vi "Shooter RPM Testing.vi"   [LabVIEW 2019]
uses:
  <vilib>/Rock Robotics/WPI/ThirdParty/REV Robotics/SPARK MAX/Typedef/Spark MAX Control Type.ctl
  Robot Global Data.vi
  <vilib>/Analysis/NI_AALPro.lvlib
types:
  T1 = typedef "WPI_MotorControlDeviceRef.ctl" = cluster{"DeviceStatus":errorcluster, "Type":T2, "PWM":cluster{"PWM Channel":T3, "DeadBand":T4}, "CAN":cluster{"Device Number":u8, "SetOutput VI Ref":variant, "GetOutput VI Ref":variant, "Enable VI Ref":variant, "Disable VI Ref":variant, "Data":variant}, "Invert":bool, "DIO PWM":cluster{"PWM \"Enable\" Channel":T3, "DIOChannel":T5, "PWM Rate":dbl}}
  T2 = typedef "WPI_MotorControlType.ctl" = enum16{"PWM", "CAN", "DIO PWM"}
  T3 = typedef "FPGA_DIOPWMChannel.ctl" = enum8{"PWM 0", "PWM 1", "PWM 2", "PWM 3", "PWM 4", "PWM 5", "PWM 6", "PWM 7", "PWM 8", "PWM 9", "PWM MXP 0", "PWM MXP 1", "PWM MXP 2", "PWM MXP 3", "PWM MXP 4", "PWM MXP 5", "PWM MXP 6", "PWM MXP 7", "PWM MXP 8", "PWM MXP 9", "Invalid"}
  T4 = typedef "WPI_PWMDeadband.ctl" = cluster{"Name":string, "maxPositivePwm":i32, "minPositivePwm":i32, "centerPwm":i32, "maxNegativePwm":i32, "minNegativePwm":i32, "angularRange":u16}
  T5 = typedef "FPGA_DIOChannel.ctl" = enum8{"DIO 0", "DIO 1", "DIO 2", "DIO 3", "DIO 4", "DIO 5", "DIO 6", "DIO 7", "DIO 8", "DIO 9", "DIO MXP 0", "DIO MXP 1", "DIO MXP 2", "DIO MXP 3", "DIO MXP 4", "DIO MXP 5", "DIO MXP 6", "DIO MXP 7", "DIO MXP 8", "DIO MXP 9", "DIO MXP 10", "DIO MXP 11", "DIO MXP 12", "DIO MXP 13", "DIO MXP 14", "DIO MXP 15", "SPI Port CS1", "SPI Port CS2", "SPI Port CS3", "SPI Port MISO", "SPI Port MOSI", "Invalid"}
  T6 = typedef "Spark MAX Control Type.ctl" = enum16{"Percent VBus", "Voltage", "Velocity", "Position", "Smart Motion", "Current", "Smart Velocity"}
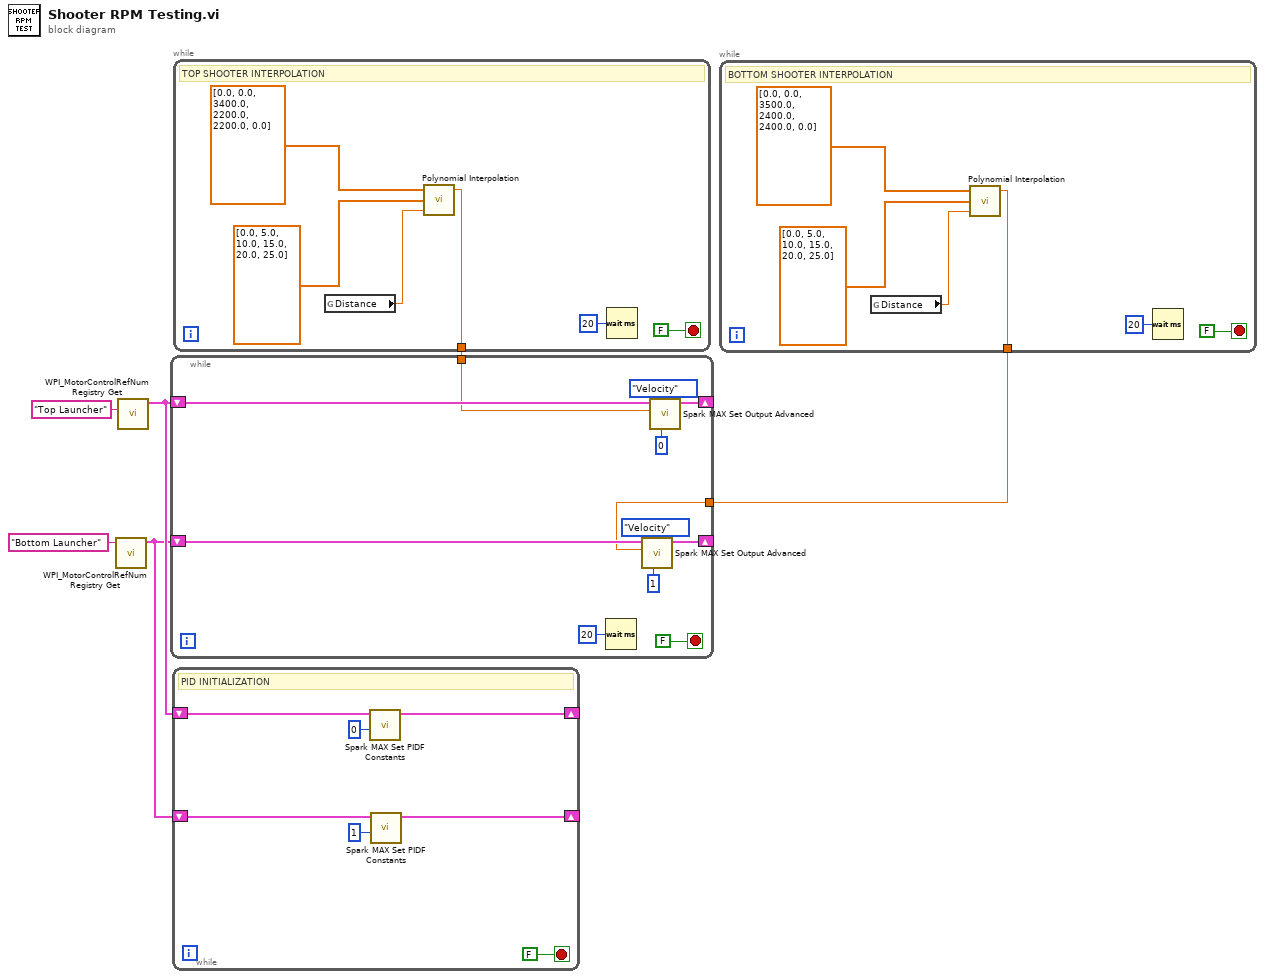
[diagram p0: block diagram]
diagram:
  n1 = call <vilib>:"WPI_MotorControlRefNum Registry Get.vi"("refnum name"="Bottom Launcher") -> ("MotorControlDevRef"=w1:T1)  [unwired: 9 in, 1 out]
  n2 = call <vilib>:"WPI_MotorControlRefNum Registry Get.vi"("refnum name"="Top Launcher") -> ("MotorControlDevRef"=w2:T1)  [unwired: 9 in, 1 out]
  n3 = while {
    shift-right: [w11] -> _
    shift-left: w2 -> [w12]
    shift-right: [w7] -> _
    shift-left: w1 -> [w8]
    stop <- FALSE stop-if-true
    # "PID INITIALIZATION"
    n4 = call <vilib>:"Spark MAX Set PIDF Constants.vi"("PIDF Slot"=0, "MotorControlDeviceRef"=w12) -> ("MotorControlDeviceRef"=w11:T1)  [unwired: 8 in, 1 out]
    n5 = call <vilib>:"Spark MAX Set PIDF Constants.vi"("PIDF Slot"=1, "MotorControlDeviceRef"=w8) -> ("MotorControlDeviceRef"=w7:T1)  [unwired: 8 in, 1 out]
  }
  n6 = while {
    tunnel: [w14] -> w5
    stop <- FALSE stop-if-true
    # "TOP SHOOTER INTERPOLATION"
    n7 = global read "Robot Global Data.vi" "Distance"() -> (w15:dbl)
    n8 = call <vilib>:"Polynomial Interpolation.vi"("x value"=w15, "X"=dbl[] [0.0, 5.0, 10.0, 15.0, 20.0, 25.0], "Y"=dbl[] [0.0, 0.0, 3400.0, 2200.0, 2200.0, 0.0]) -> ("interpolation value"=w14:dbl)  [unwired: 2 out]
    n9 = Wait (ms)(milliseconds to wait=u32 20) -> ()  [unwired: 1 out]
  }
  n10 = while {
    tunnel: [w20] -> w3
    stop <- FALSE stop-if-true
    # "BOTTOM SHOOTER INTERPOLATION"
    n11 = global read "Robot Global Data.vi" "Distance"() -> (w21:dbl)
    n12 = call <vilib>:"Polynomial Interpolation.vi"("x value"=w21, "X"=dbl[] [0.0, 5.0, 10.0, 15.0, 20.0, 25.0], "Y"=dbl[] [0.0, 0.0, 3500.0, 2400.0, 2400.0, 0.0]) -> ("interpolation value"=w20:dbl)  [unwired: 2 out]
    n13 = Wait (ms)(milliseconds to wait=u32 20) -> ()  [unwired: 1 out]
  }
  n14 = while {
    shift-right: [w36] -> _
    shift-left: w2 -> [w35]
    tunnel: w5 -> [w32]
    shift-right: [w31] -> _
    shift-left: w1 -> [w29]
    tunnel: w3 -> [w28]
    stop <- FALSE stop-if-true
    n15 = Wait (ms)(milliseconds to wait=u32 20) -> ()  [unwired: 1 out]
    n16 = call <vilib>:"Spark MAX Set Output Advanced.vi"("PIDF Slot (0)"=1, "Control Mode"=Spark_MAX_Control_Type."Velocity", "Setpoint"=w28, "MotorControlDevRef"=w29) -> ("MotorControlDevRef"=w31:T1)  [unwired: 6 in, 1 out]
    n17 = call <vilib>:"Spark MAX Set Output Advanced.vi"("PIDF Slot (0)"=0, "Control Mode"=Spark_MAX_Control_Type."Velocity", "Setpoint"=w32, "MotorControlDevRef"=w35) -> ("MotorControlDevRef"=w36:T1)  [unwired: 6 in, 1 out]
  }
